vi "get grouped data.vi"(10 "Index":i32, 11 "Full Data Set":dbl[][](array[numeric])) -> (2 "Small Group":dbl[][](array[numeric]), 3 "Large Group":dbl[][](array[numeric]))   [LabVIEW 2020]
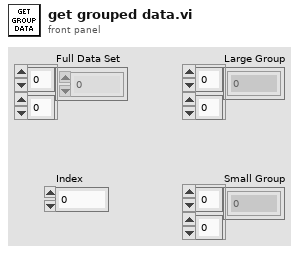
[diagram p1: front panel]
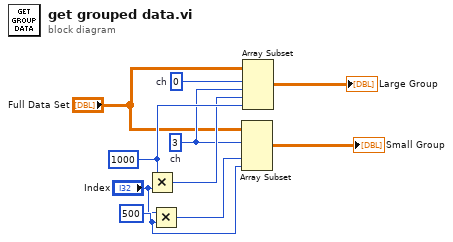
[diagram p0: block diagram]
diagram:
  w7 = 500 ("x")
  w6 = 1000 ("x")
  w3 = 3  # ch
  w2 = 0  # ch
  n1 = Multiply(x=w6, y="Index") -> (x*y=w5:i32)
  n2 = Multiply(x="Index", y=w7) -> (x*y=w8:i32)
  n3 = Array Subset(array="Full Data Set", index (row)=w3, index (col)=w8, length (col)=w7) -> (→"Small Group":dbl[][])  [unwired: 1 in]
  n4 = Array Subset(array="Full Data Set", index (row)=w2, length (row)=w3, index (col)=w5, length (col)=w6) -> (→"Large Group":dbl[][])
